vi "数据库删除.vi"(8 "error in (no error)":errorcluster caption="错误输入（无错误）") -> (0 "error out":errorcluster caption="错误输出", 2 "已发送数据":string[][](table), 3 "待发送数据":string[][](table))   [LabVIEW 2016, in "数据传输系统-03.lvlib"]
uses:
  <vilib>/Utility/sysdir.llb/System Directory Type.ctl
  <vilib>/addons/database/Connection.llb/DB Tools Open Connec (String).vi
  <vilib>/addons/database/_DB Variant To Data/Database Variant To Data.xnode
  <vilib>/addons/database/NI_Database_API.lvlib
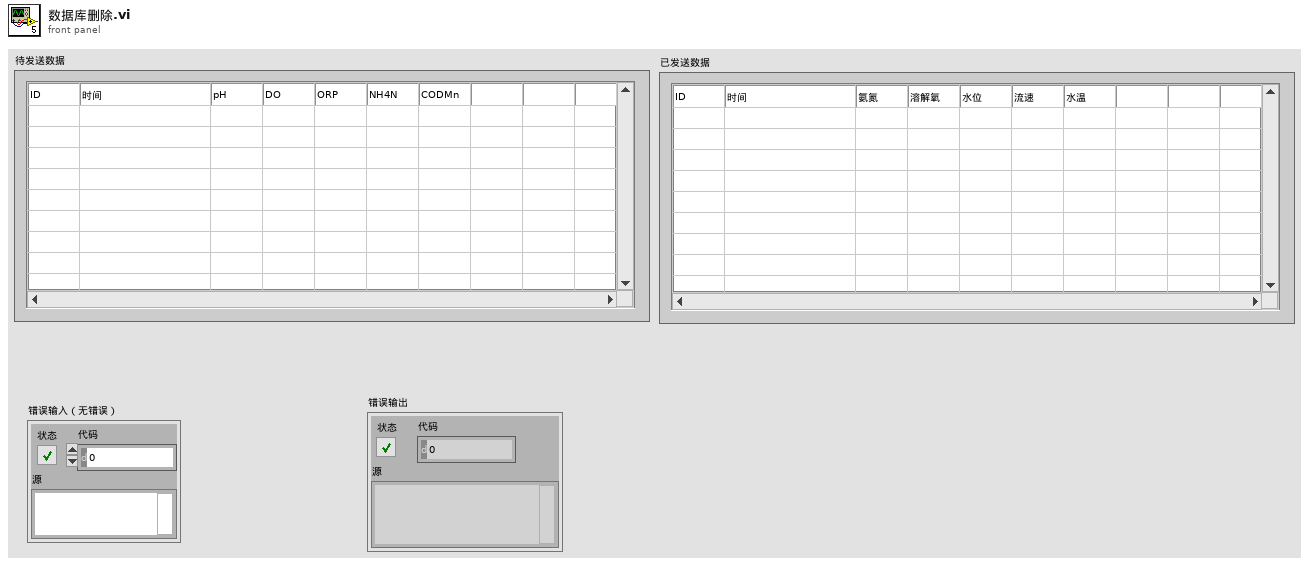
[diagram p1: front panel]
types:
  T1 = typedef "System Directory Type.ctl" = i32
  T2 = typedef "NI_Database_API.lvlib/Conn ObjectReference.ctl" = refnum<k1>
  T3 = cluster{string, string, string, string, string, string}
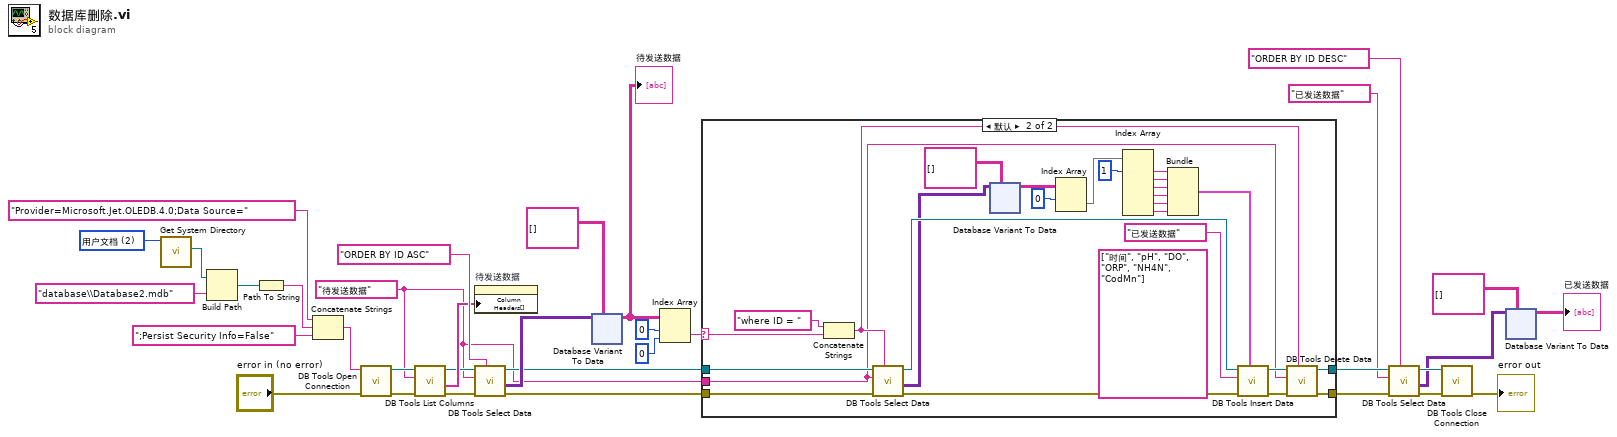
[diagram p0: block diagram]
diagram:
  w8 = T1 2 items=["用户目录"=0, "用户桌面"=1, "用户文档"=2, "用户应用程序数据"=3, "用户设置"=4, "用户临时目录"=5, "公共文档"=6, "公共应用程序数据"=7, "公共设置"=8, "公共缓存"=13, "系统核心库"=9, "系统安装库"=10, "应用程序文件"=11, "启动盘根目录"=12] ("system directory type")
  w18 = "待发送数据" ("组合框")
  n1 = call <vilib>:"Get System Directory.vi"("system directory type"=w8) -> ("system directory"=w6:path)  [unwired: 10 in]
  n2 = Build Path(base path=w6, name or relative path="database\\Database2.mdb" ("condition")) -> (appended path=w5:path)
  n3 = Path To String(path=w5) -> (string=w4:string)
  n4 = Concatenate Strings("Provider=Microsoft.Jet.OLEDB.4.0;Data Source=" ("condition"), w4, ";Persist Security Info=False" ("condition")) -> (w2:string)
  n5 = call-poly <vilib>:"DB Tools Open Connection.vi"("error in (no error)"="error in (no error)", "connection information"=w2) -> ("error out"=w28:errorcluster, "connection reference"=w26:T2)  [unwired: 6 in]
  n6 = call <vilib>:"DB Tools List Columns.vi"("error in (no error)"=w28, "table"=w18, "connection reference"=w26) -> ("error out"=w27:errorcluster, "columns"=w29:string[], "connection reference out"=w25:T2)  [unwired: 1 in, 1 out]
  n7 = property on="待发送数据" class="Tbl (严格)"("Column Headers[]"=w29) -> ()  [unwired: 2 in, 2 out]
  n8 = call <vilib>:"DB Tools Select Data.vi"("condition"="ORDER BY ID ASC", "error in (no error)"=w27, "table"=w18, "connection reference"=w25) -> ("error out"=w21:errorcluster, "data"=w34:variant[][], "connection reference out"=w19:T2)  [unwired: 2 in]
  n9 = xnode "Database Variant To Data"("database variant"=w34, "type"=string[][] []) -> ("data"=w20:string[][])  [unwired: 1 in, 1 out]
  "待发送数据" <- w20
  n10 = Index Array(array=w20, index (row)=0 ("索引 (行)"), index (col)=0 ("禁用的索引 (列)")) -> (element=w22:string)
  n11 = case shown="默认" w22 {
    selector: w22 -> [_ w61]
    tunnel: w21 -> [w35 w60]
    tunnel: w19 -> [w36 w58]
    tunnel: [w36 w38] -> w13
    tunnel: [w35 w37] -> w14
    tunnel: w18 -> [_ w40]
    frame "" {
    }
    frame Default {
      (unwired) string[] ["时间", "pH", "DO", "ORP", "NH4N", "CodMn"] ("columns")
      n12 = Concatenate Strings("where ID = " ("字符串"), w61) -> (w59:string)
      n13 = call <vilib>:"DB Tools Select Data.vi"("condition"=w59, "error in (no error)"=w60, "table"=w40, "connection reference"=w58) -> ("error out"=w54:errorcluster, "data"=w53:variant[][], "connection reference out"=w57:T2)  [unwired: 2 in]
      n14 = xnode "Database Variant To Data"("database variant"=w53, "type"=string[][] []) -> ("data"=w51:string[][])  [unwired: 1 in, 1 out]
      n15 = Index Array(array=w51, index (row)=0 ("索引 (行)")) -> (element=w49:string[])  [unwired: 1 in]
      n16 = Index Array(array=w49, index #1=1 ("索引")) -> (element #1=w47:string, element #2=w46:string, element #3=w45:string, element #4=w44:string, element #5=w43:string, element #6=w42:string)  [unwired: 5 in]
      n17 = Bundle(w47, w46, w45, w44, w43, w42) -> (w41:T3)  [unwired: 1 in]
      n18 = call <vilib>:"DB Tools Insert Data.vi"("data"=w41, "error in (no error)"=w54, "table"="已发送数据" ("组合框"), "connection reference"=w57) -> ("error out"=w56:errorcluster, "connection reference out"=w55:T2)  [unwired: 6 in]
      n19 = call <vilib>:"DB Tools Delete Data.vi"("condition"=w59, "error in (no error)"=w56, "table"=w40, "connection reference"=w55) -> ("error out"=w37:errorcluster, "connection reference out"=w38:T2)  [unwired: 6 in]
    }
  }
  n20 = call <vilib>:"DB Tools Select Data.vi"("condition"="ORDER BY ID DESC", "error in (no error)"=w14, "table"="已发送数据" ("组合框"), "connection reference"=w13) -> ("error out"=w15:errorcluster, "data"=w10:variant[][], "connection reference out"=w12:T2)  [unwired: 2 in]
  n21 = call <vilib>:"DB Tools Close Connection.vi"("error in (no error)"=w15, "connection reference"=w12) -> ("error out"=→"error out":errorcluster)  [unwired: 5 in]
  n22 = xnode "Database Variant To Data"("database variant"=w10, "type"=string[][] []) -> ("data"=→"已发送数据":string[][])  [unwired: 1 in, 1 out]
